vi "bufferSelect.vi"(0 "SPI Config In":T1) -> (1 "SPI Config Out":T1, 2 "Buffer":cluster{"Buffer Num":u8, "Buffer Addr":u8})   [LabVIEW 2019]
uses:
  SPI/SPI Config.ctl
  <vilib>/rvi/Emulation/niFpgaGetClockAttributes.vi
  <vilib>/rvi/Emulation/niFpgaSctlEmulationGetInTimedLoop.vi
  <vilib>/rvi/Emulation/niFpgaEmulationReportErrorSimple.vi
  <vilib>/rvi/Emulation/niFpgaCriticalErrorInLSC.vi
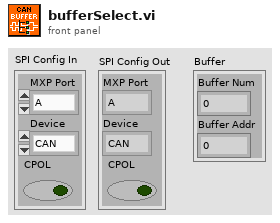
[diagram p1: front panel]
types:
  T1 = typedef "SPI Config.ctl" = cluster{"MXP Port":enum16{"A", "B"}, "Device":enum16{"CAN", "ENC", "IMU1", "IMU2"}, "CPOL":bool}
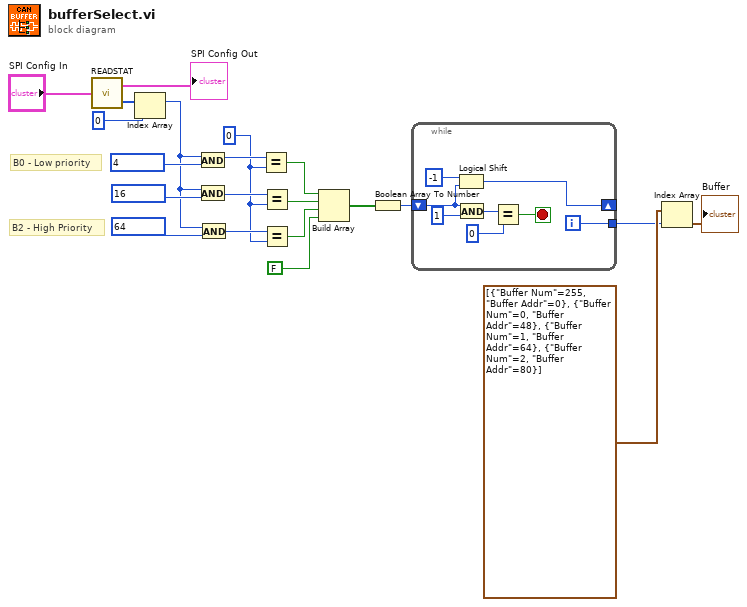
[diagram p0: block diagram]
diagram:
  w15 = u8 0 ("y")
  # "B2 - High Priority"
  # "B0 - Low priority"
  n1 = call "READSTAT.vi"("SPI Config In"="SPI Config In") -> ("SPI Config Out"=→"SPI Config Out":T1, "Frames Read"=w8:u8[])
  n2 = Index Array(array=w8, index=0) -> (element=w7:u8)
  n3 = And(x=w7, y=u8 4) -> (x .and. y?=w18:u8)
  n4 = And(x=w7, y=u8 16) -> (x .and. y?=w17:u8)
  n5 = And(x=w7, y=u8 64) -> (x .and. y?=w16:u8)
  n6 = Equal?(x=w18, y=w15) -> (x = y?=w14:bool)
  n7 = Equal?(x=w17, y=w15) -> (x = y?=w13:bool)
  n8 = Equal?(x=w16, y=w15) -> (x = y?=w12:bool)
  n9 = Build Array(w14, w13, w12, FALSE ("element")) -> (w5:bool[])
  n10 = Boolean Array To Number(Boolean array=w5) -> (number=w4:u8)
  n11 = while {
    shift-right: [w23] -> _
    shift-left: w4 -> [w24]
    tunnel: [w22] -> w2
    i -> [w22]
    stop <- w26 stop-if-true
    n12 = Logical Shift(y=i16 -1, x=w24) -> (x << y=w23:u8)
    n13 = And(x=w24, y=u8 1) -> (x .and. y?=w28:u8)
    n14 = Equal?(x=w28, y=u8 0) -> (x = y?=w26:bool)
  }
  n15 = Index Array(array=cluster{"Buffer Num":u8, "Buffer Addr":u8}[] [{"Buffer Num"=255, "Buffer Addr"=0}, {"Buffer Num"=0, "Buffer Addr"=48}, {"Buffer Num"=1, "Buffer Addr"=64}, {"Buffer Num"=2, "Buffer Addr"=80}], index=w2) -> (element=→"Buffer":cluster{"Buffer Num":u8, "Buffer Addr":u8})
